vi "Autoshift Loop.vi"(9 "Turn Power":dbl) -> (2 "Shift?":bool)   [LabVIEW 2017]
uses:
  Robot Global Data.vi
  <vilib>/express/express arith-compare/Formula/XNode/ExpressFormulaBlockNode.xnode
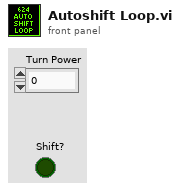
[diagram p1: front panel]
types:
  T1 = typedef "Dashboard Control Data.ctl" = cluster{"Drivetrain Settings Cluster":T2, "Intake Presets":T7, "Elevator Settings Cluster":T8, "Drivetrain Encoder Values":T10, "Auton Chooser":T11, "Auton Presets":cluster{"Start Position":dbl}, "Elevator Encoder Values":T12, "Pressure M":dbl, "Pressure B":dbl, "Zero All?":bool, "Enable Vision":bool}
  T2 = typedef "Drivetrain Settings Cluster.ctl" = cluster{"Gyro Steer PID Gains":T3, "Distance Drive PID Gains":T3, "Drive Tolerance":dbl, "Gyro Tolerance":dbl, "Gyro Output":dbl, "Distance Output":dbl, "Y Power Multiplier":dbl, "Turn Power Multiplier":dbl, "Creep Rate":dbl, "Encoder Reset":bool, "DT Mode Modifier":enum16{"None, Default", "Cube", "Square"}, "Left Encoder Tick Constant":dbl, "Right Encoder Tick Constant":dbl, "Shift Speed":dbl, "Zero Gyro":bool, "Y min":dbl, "Y max":dbl, "X min":dbl, "X max":dbl, "Finish Velocity":dbl, "Anti-Tip Settings":T4, "Trapezoidal Settings":T5, "Turning, Don't Shift":dbl, "Shift time":dbl}
  T3 = typedef "PID Gains Cluster.ctl" = cluster{"Proportional Gain":dbl, "Integral Time":dbl, "Derivative Time":dbl}
  T4 = typedef "Anti-Tip Settings.ctl" = cluster{"Pitch Tip Constant":dbl, "Wheel Diameter":dbl, "Gearbox Reduction":dbl, "Motor Count":dbl, "Mass of Robot":dbl, "Almost Tip Constant":dbl, "Dist to CG":dbl}
  T5 = typedef "Trapezoidal Settings.ctl" = cluster{"1st Gear Reduction":dbl, "2nd Gear Reduction":dbl, "Maximum RPM":dbl, "1st Gear PVA Gains":T6, "2nd Gear PVA Gains":T6, "Wheel Radius":dbl, "Mass of the Wheel":dbl, "Number of Motors":dbl, "Velocity Tolerance":dbl, "Cruise Time (ms)":dbl, "Efficiency":dbl}
  T6 = typedef "PVA Gains.ctl" = cluster{"Positional Gain":dbl, "Velocity Gain":dbl, "Acceleration Gain":dbl}
  T7 = typedef "Intake Presets.ctl" = cluster{"Idle Angle":dbl, "Mid Angle":dbl, "Low Angle":dbl, "Outtake Power":dbl, "Intake Power":dbl, "Unstuck":dbl, "Angle Tolerance":dbl, "Max Angle":dbl, "Max Current":dbl, "Current Trip Time":dbl, "Reset Encoder?":bool, "Encoder Scale":dbl, "PID gains":cluster{"proportional gain (Kc)":dbl, "integral time (Ti, min)":dbl, "derivative time (Td, min)":dbl}, "output range":cluster{"output high":dbl, "output low":dbl}, "IR Constant Pull Rate":dbl, "Shoot Angle":dbl, "Shoot High":dbl, "Manual Limit":dbl}
  T8 = typedef "Elevator Settings Cluster.ctl" = cluster{"Ground Height":dbl, "Switch Height":dbl, "Scale High Height ":dbl, "Scale Low Height":dbl, "Elevator PID Gains":T9, "Elevator Tolerance":dbl, "Reset Encoders":bool, "Encoder Scale":dbl, "Max Height":dbl, "Mid Height":dbl, "output range":cluster{"output high":dbl, "output low":dbl}, "Upper Slow Down Tolerance":dbl, "Tick Constant":dbl, "Tip Constant":dbl, "Slow Down Multiplier":dbl, "Almost Tip Constant":dbl, "Bottom Trip Offset":dbl, "Lower Slow Down Tolerance":dbl, "Cruise Velocity":dbl, "Max Acceleration":dbl, "Feed Forward":dbl}
  T9 = typedef "PID Gains.ctl" = cluster{"proportional gain (Kc)":dbl, "integral time (Ti, min)":dbl, "derivative time (Td, min)":dbl}
  T10 = typedef "DT Encoder Values.ctl" = cluster{"Left Encoder":cluster{"Distance":dbl, "Speed":dbl, "Tick":dbl}, "Right Encoder":cluster{"Distance":dbl, "Speed":dbl, "Tick":dbl}}
  T11 = typedef "Auton Chooser.ctl" = cluster{"Left":bool, "Center":bool, "Right":bool, "Scale":bool, "Both":bool, "Switch":bool, "Test":bool, "No Script":bool, "Drive PID":bool, "Elevator PID":bool, "Gyro PID":bool, "Drive Forward":bool, "cross front":bool, "Near":bool, "Far":bool, "1 Plus 1":bool, "2 Scale":bool, "2 Switch":bool, "cross behind":bool, "Pick up 2nd cube":bool, "No cross if cross":bool}
  T12 = typedef "Elevator Encoder Values.ctl" = cluster{"Encoder Values":cluster{"Distance":dbl, "Speed":dbl, "Tick":dbl}}
  T13 = typedef "Drivetrain Status Cluster.ctl" = cluster{"Throttle (Y)":dbl, "Steer (X)":dbl, "Drivetrain Mode":T14, "Brake?":bool, "Distance Drive Complete?":bool, "PID Drive Complete?":bool, "Creep Mode?":bool, "Gyro Steer Complete?":bool, "Gyro":dbl, "Heading Target":dbl, "Distance Target":dbl, "2nd Gear":bool, "Drivetrain Encoder Values":T10, "Left Motor Power":dbl, "Right Motor Power":dbl, "Auto Shift States":T15}
  T14 = typedef "Drivetrain Mode.ctl" = enum16{"Manual w/ Autoshift", "Trapezoidal Motion", "Manual", "Gyro Steer", "PID Drive", "Distance Drive", "Autonomous"}
  T15 = typedef "Auto Shift States.ctl" = enum16{"First Gear", "Second Gear"}
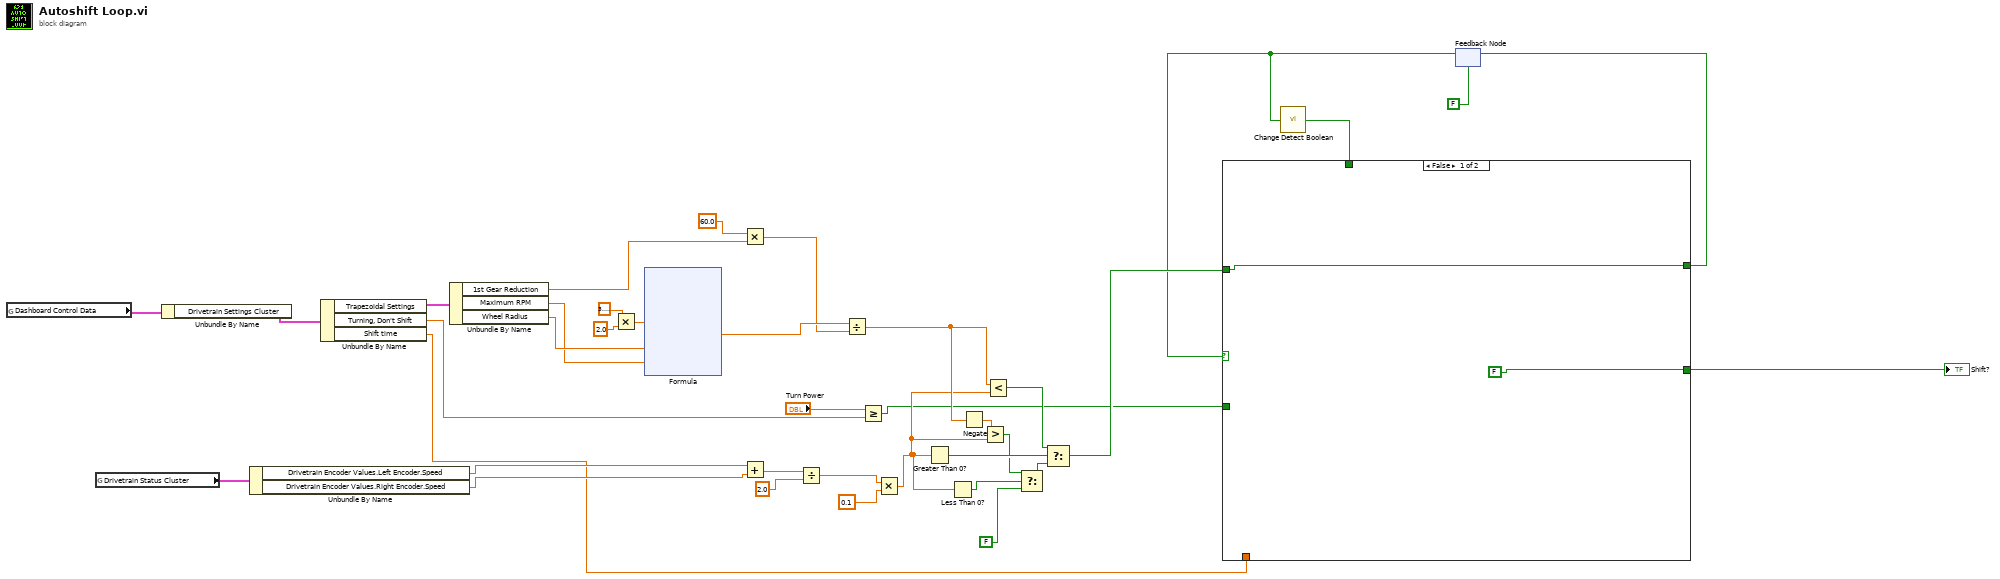
[diagram p0: block diagram]
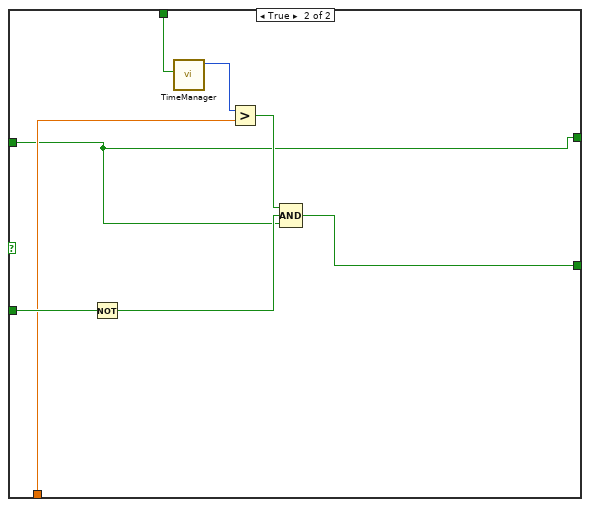
[diagram p2: hidden frame]
diagram:
  n1 = global read "Robot Global Data.vi" "Dashboard Control Data"() -> (w38:T1)
  n2 = global read "Robot Global Data.vi" "Drivetrain Status Cluster"() -> (w20:T13)
  n3 = Unbundle By Name(w38) -> ("Drivetrain Settings Cluster"=w37:T2)
  n4 = Unbundle By Name(w20) -> ("Drivetrain Encoder Values.Left Encoder.Speed"=w19:dbl, "Drivetrain Encoder Values.Right Encoder.Speed"=w18:dbl)
  n5 = Unbundle By Name(w37) -> ("Trapezoidal Settings"=w30:T5, "Turning, Don't Shift"=w31:dbl, "Shift time"=w1:dbl)
  n6 = Unbundle By Name(w30) -> ("1st Gear Reduction"=w24:dbl, "Maximum RPM"=w25:dbl, "Wheel Radius"=w26:dbl)
  n7 = Multiply(x=3.141592653589793, y=2.0) -> (x*y=w27:dbl)
  n8 = xnode "Formula"("2PI"=w27, "Wheel Radius"=w26, "Max RPM"=w25) -> ("Result"=w22:dbl)  [unwired: 1 in, 1 out]
  n9 = Multiply(x=60.0, y=w24) -> (x*y=w21:dbl)
  n10 = Add(x=w19, y=w18) -> (x+y=w36:dbl)
  n11 = Divide(x=w36, y=2.0) -> (x/y=w34:dbl)
  n12 = Divide(x=w22, y=w21) -> (x/y=w14:dbl)
  n13 = Greater Or Equal?(x="Turn Power", y=w31) -> (x >= y?=w2:bool)
  n14 = Multiply(x=w34, y=0.1) -> (x*y=w11:dbl)
  n15 = Greater Than 0?(x=w11) -> (x > 0?=w17:bool)
  n16 = Less Than 0?(x=w11) -> (x < 0?=w15:bool)
  n17 = Negate(x=w14) -> (-x=w13:dbl)
  n18 = Greater?(x=w13, y=w11) -> (0:w12:bool)
  n19 = Less?(x=w14, y=w11) -> (x < y?=w16:bool)
  n20 = Select(t=w12, s=w15, f=FALSE) -> (s? t:f=w9:bool)
  n21 = Select(t=w16, s=w17, f=w9) -> (s? t:f=w8:bool)
  n22 = feedback #1(FALSE) -> (w4:bool)
  n23 = call "Change Detect Boolean.vi"("In"=w4) -> ("Changed?"=w3:bool)
  n24 = case shown="False" w4 {
    tunnel: w8 -> [w40 w41]
    tunnel: [w40 w41] -> w6
    tunnel: [FALSE w42] -> w5
    tunnel: w3 -> [_ w48]
    tunnel: w2 -> [_ w46]
    tunnel: w1 -> [_ w43]
    frame False {
    }
    frame True {
      n25 = Not(x=w46) -> (.not. x?=w44:bool)
      n26 = call "TimeManager.vi"("Reset?"=w48) -> ("Time Since Reset"=w47:u32)  [unwired: 9 in, 1 out]
      n27 = Greater?(x=w47, y=w43) -> (0:w45:bool)
      n28 = Compound Arithmetic op=AND(w45, w44, w41) -> (w42:bool)
    }
  }
  "Shift?" <- w5
  n29 = feedback-in #1(w6) -> ()
